vi "lab_3.vi"() -> ()   [LabVIEW 2015]
uses:
  <vilib>/Analysis/Matrix/NI_Matrix.lvlib
  <vilib>/Analysis/Matrix/Numeric/Conversions/Matrix To Array - RM.vi
  ProcessingDLL4/x64/Debug/ProcessingDLL4.dll
panel:
  out "Result":picture
  in  "Method":u16(ring) items=["Nothing", "Sub VI", "DLL"]
  in  "Stop":bool
  in  "Kernel Dim":u8(slide)=3 min=3 max=9 step=1 scale=3.0..9.0
  in  "Kernel":dbl[][](array[numeric])
  out "Original":picture
  in  "Path":path
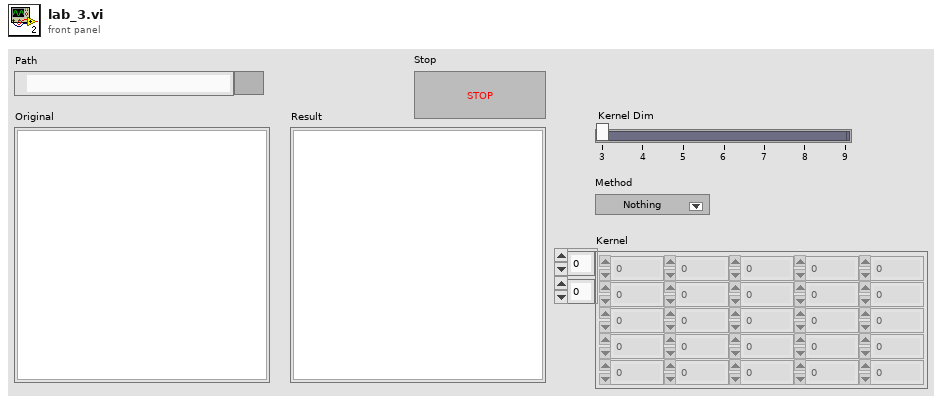
[diagram p1: front panel]
types:
  T1 = typedef "LVBoundsTypeDef.ctl" = cluster{"Width":u32, "Height":u32}
  T2 = typedef "imagedata.ctl" = cluster{"image type":i32, "image depth":i32, "image":u8[], "mask":u8[], "colors":u32[], "Rectangle":cluster{"left":i16, "top":i16, "right":i16, "bottom":i16}}
  T3 = typedef "NI_Matrix.lvlib/RealMatrix.ctl" = dbl[][]
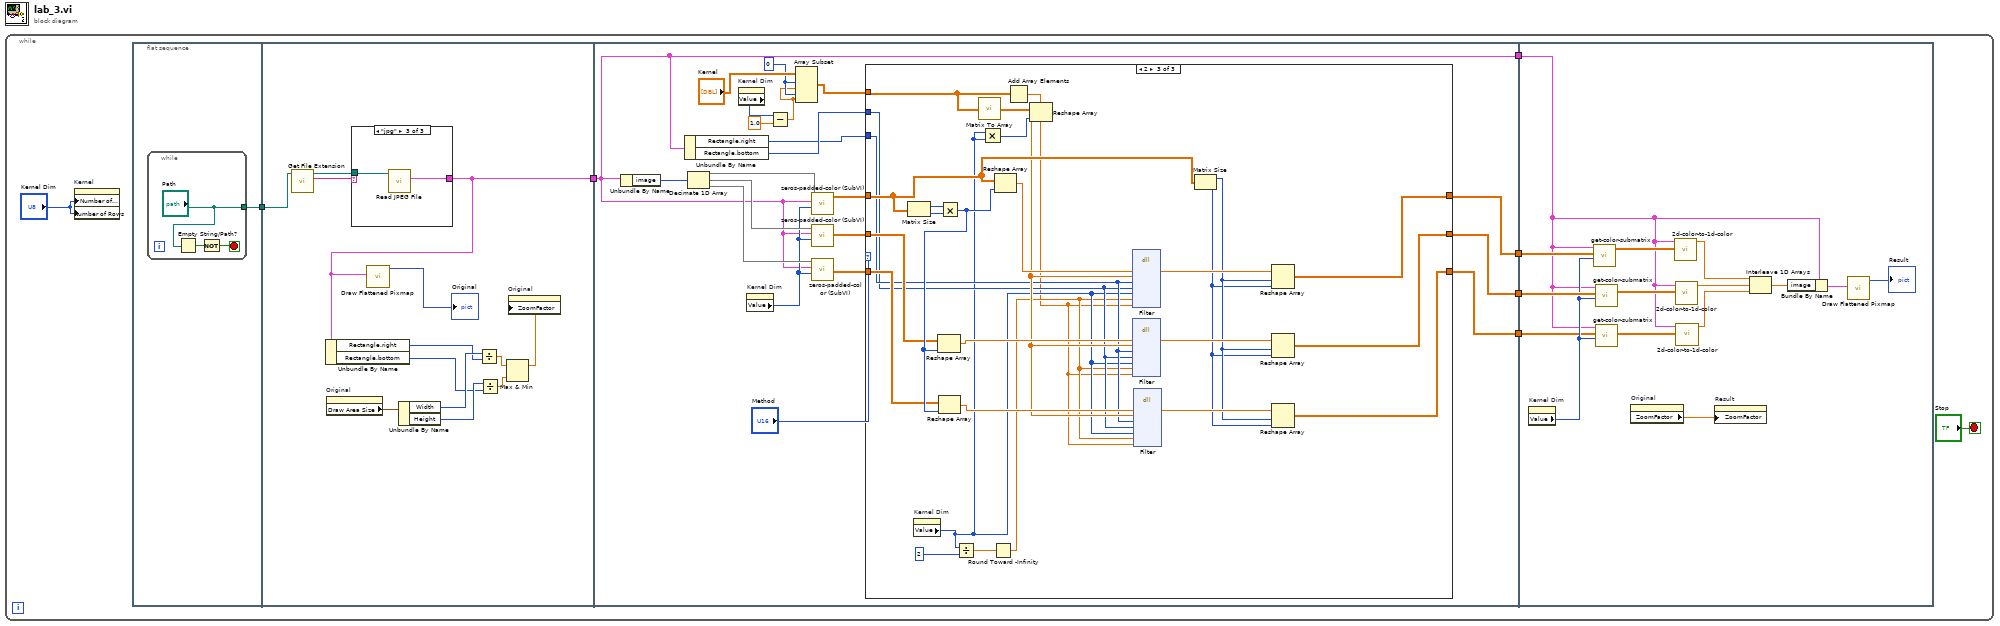
[diagram p0: block diagram]
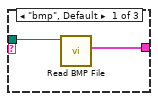
[diagram p2: hidden frame]
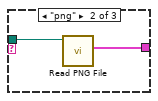
[diagram p3: hidden frame]
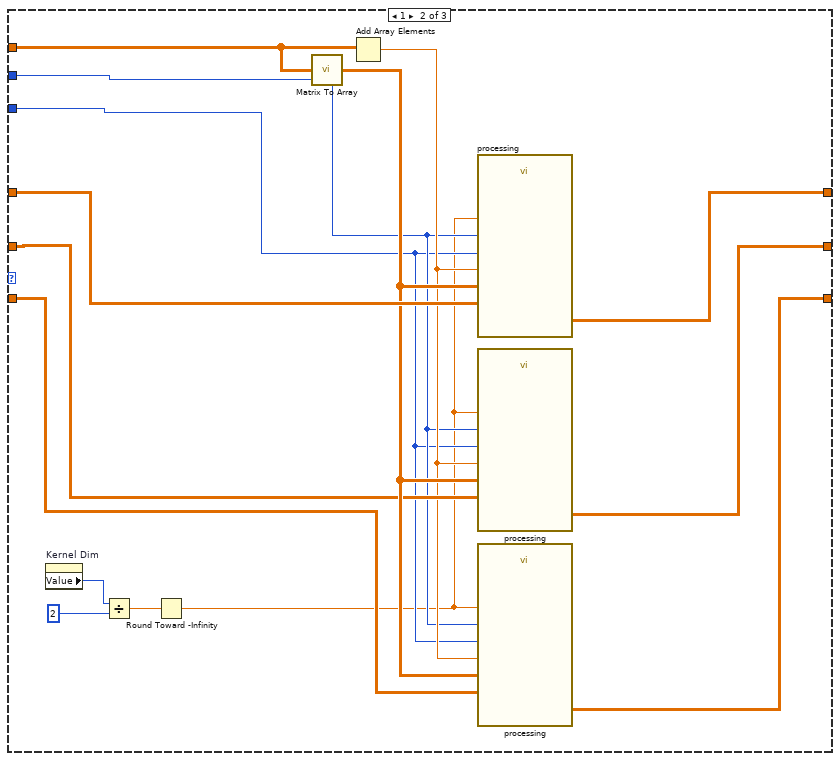
[diagram p5: hidden frame]
diagram:
  n1 = while {
    stop <- "Stop" stop-if-true
    n2 = property on="Kernel" class="Arr (strict)"("Number of Columns"="Kernel Dim", "Number of Rows"="Kernel Dim") -> ()  [unwired: 2 in, 2 out]
    n3 = flat-sequence {
      tunnel: [w9] -> w2
      tunnel: [w16] -> w7
      tunnel: w2 -> [w13]
      tunnel: w7 -> [w40]
      tunnel: [w40] -> w6
      tunnel: [w46] -> w5
      tunnel: [w44] -> w4
      tunnel: [w42] -> w3
      tunnel: w6 -> [w99]
      tunnel: w5 -> [w113]
      tunnel: w4 -> [w112]
      tunnel: w3 -> [w110]
      frame #0 {
        n4 = while {
          tunnel: ["Path"] -> w9
          stop <- w11 stop-if-true
          n5 = Empty String/Path?(string/path="Path") -> (empty?=w12:bool)
          n6 = Not(x=w12) -> (.not. x?=w11:bool)
        }
      }
      frame #1 {
        n7 = call <vilib>:"Get File Extension.vi"("file"=w13) -> ("lowercase file extension"=w14:string, "dup file"=w15:path)  [unwired: 6 in, 3 out]
        n8 = property on="Original" class="Pict"() -> ("Draw Area Size"=w24:T1)  [unwired: 2 in, 2 out]
        n9 = case shown="\"jpg\"" w14 {
          tunnel: w15 -> [w27 w29 w31]
          tunnel: [w26 w28 w30] -> w16
          frame "bmp", Default {
            n10 = call <vilib>:"Read BMP File.vi"("path to BMP file"=w27) -> ("image data"=w26:T2)  [unwired: 8 in, 2 out]
          }
          frame "png" {
            n11 = call <vilib>:"Read PNG File.vi"("path to PNG file"=w29) -> ("image data"=w28:T2)  [unwired: 8 in, 2 out]
          }
          frame "jpg" {
            n12 = call <vilib>:"Read JPEG File.vi"("path to JPEG file"=w31) -> ("image data"=w30:T2)  [unwired: 8 in, 2 out]
          }
        }
        n13 = Unbundle By Name(w16) -> ("Rectangle.right"=w21:i16, "Rectangle.bottom"=w20:i16)
        n14 = call <vilib>:"Draw Flattened Pixmap.vi"("image data"=w16) -> ("new picture"=→"Original":picture)  [unwired: 8 in]
        n15 = Unbundle By Name(w24) -> ("Width"=w23:u32, "Height"=w22:u32)
        n16 = Divide(x=w23, y=w21) -> (x/y=w19:dbl)
        n17 = Divide(x=w22, y=w20) -> (x/y=w17:dbl)
        n18 = Max & Min(x=w19, y=w17) -> (max(x,y)=w18:dbl)  [unwired: 1 out]
        n19 = property on="Original" class="Pict"("ZoomFactor"=w18) -> ()  [unwired: 2 in, 2 out]
      }
      frame #2 {
        w36 = 0 ("row 1")
        n20 = Unbundle By Name(w40) -> ("image"=w52:u8[])
        n21 = Unbundle By Name(w40) -> ("Rectangle.right"=w38:i16, "Rectangle.bottom"=w39:i16)
        n22 = Decimate 1D Array(w52) -> (w51:u8[], w50:u8[], w49:u8[])
        n23 = property on="Kernel Dim" class="Slide (strict)"() -> ("Value"=w33:u8)  [unwired: 2 in, 2 out]
        n24 = property on="Kernel Dim" class="Slide (strict)"() -> ("Value"=w48:u8)  [unwired: 2 in, 2 out]
        n25 = Subtract(x=w33, y=1.0) -> (x-y=w32:dbl)
        n26 = Array Subset(array="Kernel", index (row)=w36, length (row)=w32, index (col)=w36, length (col)=w32) -> (w35:dbl[][])
        n27 = call "zeros-padded-color (SubVI).vi"("Value"=w48, "image data"=w40, "Array"=w51) -> ("Real Matrix"=w45:T3)  [unwired: 8 in]
        n28 = call "zeros-padded-color (SubVI).vi"("Value"=w48, "image data"=w40, "Array"=w50) -> ("Real Matrix"=w43:T3)  [unwired: 8 in]
        n29 = call "zeros-padded-color (SubVI).vi"("Value"=w48, "image data"=w40, "Array"=w49) -> ("Real Matrix"=w41:T3)  [unwired: 8 in]
        n30 = case shown="2" "Method" {
          tunnel: [w55 w67 w94] -> w46
          tunnel: w45 -> [w55 w68 w90]
          tunnel: [w54 w61 w83] -> w44
          tunnel: w43 -> [w54 w64 w80]
          tunnel: [w53 w60 w82] -> w42
          tunnel: w41 -> [w53 w63 w79]
          tunnel: w39 -> [_ w58 w74]
          tunnel: w35 -> [_ w59 w98]
          tunnel: w38 -> [_ w57 w75]
          frame 0, Default {
          }
          frame 1 {
            n31 = property on="Kernel Dim" class="Slide (strict)"() -> ("Value"=w66:u8)  [unwired: 2 in, 2 out]
            n32 = Divide(x=w66, y=u8 2) -> (x/y=w70:dbl)
            n33 = Round Toward -Infinity(1:w70) -> (0:w56:dbl)
            n34 = call-poly <vilib>:"Matrix To Array.vi"("Real Matrix"=w59) -> ("Real 2D Array"=w65:dbl[][])
            n35 = Add Array Elements(numeric array=w59) -> (sum=w62:dbl)
            n36 = call "processing.vi"("Kernel div"=w56, "Color channel"=w68, "Kernel"=w65, "Columns"=w57, "Rows"=w58, "Div"=w62) -> ("Result"=w67:T3)  [unwired: 5 in]
            n37 = call "processing.vi"("Kernel div"=w56, "Color channel"=w64, "Kernel"=w65, "Columns"=w58, "Rows"=w57, "Div"=w62) -> ("Result"=w61:T3)  [unwired: 5 in]
            n38 = call "processing.vi"("Kernel div"=w56, "Color channel"=w63, "Kernel"=w65, "Columns"=w58, "Rows"=w57, "Div"=w62) -> ("Result"=w60:T3)  [unwired: 5 in]
          }
          frame 2 {
            n39 = Matrix Size(0:w90) -> (1:w92:i32, 2:w91:i32)
            n40 = property on="Kernel Dim" class="Slide (strict)"() -> ("Value"=w73:u8)  [unwired: 2 in, 2 out]
            n41 = Multiply(x=w92, y=w91) -> (x*y=w81:i32)
            n42 = Reshape Array(w80, w81) -> (w78:dbl[])
            n43 = Reshape Array(w79, w81) -> (w77:dbl[])
            n44 = Divide(x=w73, y=u8 2) -> (x/y=w97:dbl)
            n45 = call-poly <vilib>:"Matrix To Array.vi"("Real Matrix"=w98) -> ("Real 2D Array"=w95:dbl[][])
            n46 = Multiply(x=w73, y=w73) -> (x*y=w93:u8)
            n47 = Round Toward -Infinity(1:w97) -> (0:w72:dbl)
            n48 = Reshape Array(w90, w81) -> (w89:dbl[])
            n49 = Add Array Elements(numeric array=w98) -> (sum=w71:dbl)
            n50 = Reshape Array(w95, w93) -> (w76:dbl[])
            n51 = dll-call lib="H:/11 sem/ProcessingDLL4/x64/Debug/ProcessingDLL4.dll" fn="Filter"("image_data"=w89, "image_kernel"=w76, "rows"=w75, "columns"=w74, "kernel_dim"=w73, "kernel_div"=w72, "div"=w71) -> ("image_data"=w88:dbl[])  [unwired: 10 in, 2 out]
            n52 = dll-call lib="H:/11 sem/ProcessingDLL4/x64/Debug/ProcessingDLL4.dll" fn="Filter"("image_data"=w78, "image_kernel"=w76, "rows"=w75, "columns"=w74, "kernel_dim"=w73, "kernel_div"=w72, "div"=w71) -> ("image_data"=w86:dbl[])  [unwired: 10 in, 2 out]
            n53 = dll-call lib="H:/11 sem/ProcessingDLL4/x64/Debug/ProcessingDLL4.dll" fn="Filter"("image_data"=w77, "image_kernel"=w76, "rows"=w75, "columns"=w74, "kernel_dim"=w73, "kernel_div"=w72, "div"=w71) -> ("image_data"=w87:dbl[])  [unwired: 10 in, 2 out]
            n54 = Matrix Size(0:w90) -> (1:w85:i32, 2:w84:i32)
            n55 = Reshape Array(w88, w85, w84) -> (w94:dbl[][])
            n56 = Reshape Array(w86, w85, w84) -> (w83:dbl[][])
            n57 = Reshape Array(w87, w85, w84) -> (w82:dbl[][])
          }
        }
      }
      frame #3 {
        n58 = property on="Kernel Dim" class="Slide (strict)"() -> ("Value"=w111:u8)  [unwired: 2 in, 2 out]
        n59 = call "get-color-submatrix.vi"("Value"=w111, "Real Matrix in"=w113, "image data"=w99) -> ("Real Matrix out"=w105:T3)  [unwired: 8 in]
        n60 = call "get-color-submatrix.vi"("Value"=w111, "Real Matrix in"=w112, "image data"=w99) -> ("Real Matrix out"=w104:T3)  [unwired: 8 in]
        n61 = call "get-color-submatrix.vi"("Value"=w111, "Real Matrix in"=w110, "image data"=w99) -> ("Real Matrix out"=w103:T3)  [unwired: 8 in]
        n62 = property on="Original" class="Pict"() -> ("ZoomFactor"=w106:sgl)  [unwired: 2 in, 2 out]
        n63 = call "2d-color-to-1d-color.vi"("Real Matrix in"=w105, "image data"=w99) -> ("Real Matrix out 2"=w102:dbl[])  [unwired: 9 in]
        n64 = call "2d-color-to-1d-color.vi"("Real Matrix in"=w104, "image data"=w99) -> ("Real Matrix out 2"=w101:dbl[])  [unwired: 9 in]
        n65 = call "2d-color-to-1d-color.vi"("Real Matrix in"=w103, "image data"=w99) -> ("Real Matrix out 2"=w100:dbl[])  [unwired: 9 in]
        n66 = property on="Result" class="Pict"("ZoomFactor"=w106) -> ()  [unwired: 2 in, 2 out]
        n67 = Interleave 1D Arrays(w102, w101, w100) -> (w109:dbl[])
        n68 = Bundle By Name(cluster=w99, "image"=w109) -> (w108:T2)
        n69 = call <vilib>:"Draw Flattened Pixmap.vi"("image data"=w108) -> ("new picture"=→"Result":picture)  [unwired: 8 in]
      }
    }
  }
